vi "Obtain list values.vi"(8 "error in (no error)":errorcluster, 10 "index (row)":i32, 11 "Nestle_Actor in":refnum<class "Nestle_Actor.lvclass">) -> (0 "error out":errorcluster, 3 "Nestle_Actor out":refnum<class "Nestle_Actor.lvclass">)   [LabVIEW 2019, in "Nestle_Actor.lvlib" / "Nestle_Actor.lvclass"]
uses:
  Nestle_Actor.lvclass
  C:/Program Files/National Instruments/LabVIEW 2019/vi.lib/ActorFramework/Actor/Actor.lvclass
  <vilib>/ActorFramework/Actor/Actor.lvclass/Actor.ctl
  Nestle_Actor.lvclass/Nestle_Actor.ctl
  UI Actor Messages/Update_buy_values Msg/Update_buy_values Msg.lvclass/Update_buy_values Msg.ctl
  <vilib>/ActorFramework/Message Enqueuer/Message Enqueuer.lvclass/Message Enqueuer.ctl
  <vilib>/ActorFramework/Message Enqueuer/Enqueue.vi
  UI Actor Messages/Update_buy_values Msg/Update_buy_values Msg.lvclass
  C:/Program Files/National Instruments/LabVIEW 2019/vi.lib/ActorFramework/Message/Message.lvclass
  <vilib>/ActorFramework/Message Priority Queue/Priority Enqueue.vi
  <vilib>/ActorFramework/Actor/Actor.lvclass
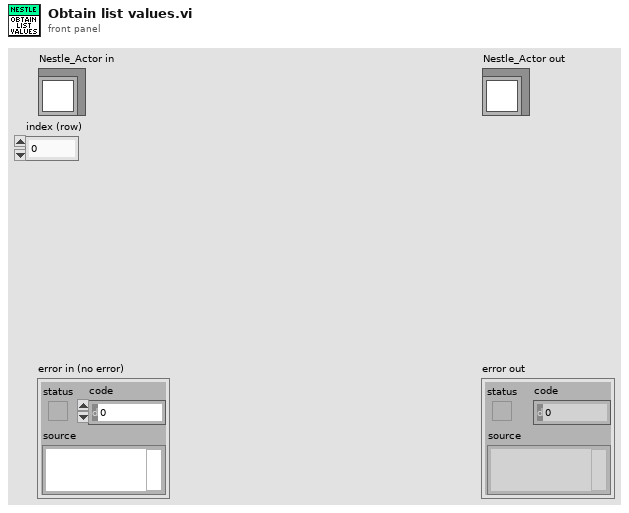
[diagram p1: front panel]
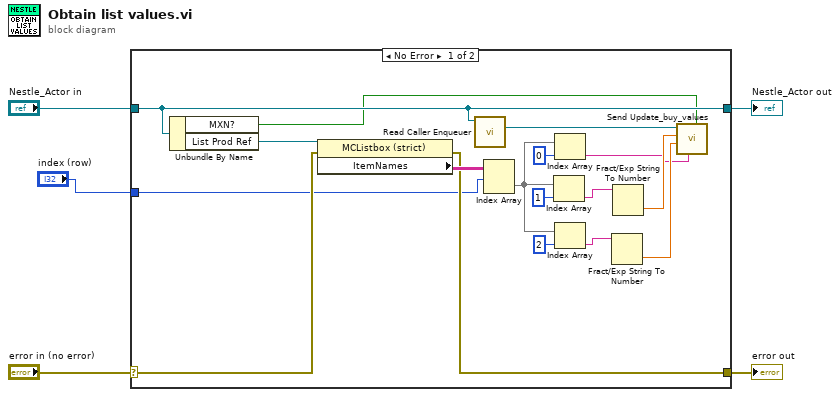
[diagram p0: block diagram]
diagram:
  n1 = case shown="No Error" "error in (no error)" {
    selector: "error in (no error)" -> [w10 w24]
    tunnel: [w9 w24] -> w4
    tunnel: [w8 w23] -> w2
    tunnel: "Nestle_Actor in" -> [w8 w23]
    tunnel: "index (row)" -> [w7 _]
    frame No Error {
      n2 = Unbundle By Name(w8) -> ("MXN?"=w6:bool, "List Prod Ref"=w11:refnum<vi>)
      n3 = property class="MCListbox (strict)"(reference=w11, error in=w10) -> (error out=w9:errorcluster, "ItemNames"=w15:string[][])  [unwired: 1 out]
      n4 = call <vilib>:"Read Caller Enqueuer.vi"("Actor"=w8) -> ("Caller Enqueuer"=w22:refnum<class "Message Enqueuer.lvclass">)  [unwired: 10 in]
      n5 = Index Array(array=w15, index (row)=w7) -> (element=w16:string[])  [unwired: 1 in]
      n6 = Index Array(array=w16, index=1) -> (element=w17:string)
      n7 = Index Array(array=w16, index=0) -> (element=w19:string)
      n8 = Index Array(array=w16, index=2) -> (element=w18:string)
      n9 = Fract/Exp String To Number(string=w18) -> (number=w20:dbl)  [unwired: 3 in, 1 out]
      n10 = Fract/Exp String To Number(string=w17) -> (number=w21:dbl)  [unwired: 3 in, 1 out]
      n11 = call "Send Update_buy_values.vi"("MXN?"=w6, "Producto"=w19, "Cantidad"=w20, "Precio"=w21, "Message Enqueuer"=w22) -> ()  [unwired: 5 in, 2 out]
    }
    frame Error {
    }
  }
  "error out" <- w4
  "Nestle_Actor out" <- w2
